vi "Close Log.vi"(0 "reference in":refnum<class "Result Logger.lvclass">, 5 "error in (no error)":errorcluster) -> (14 "reference out":refnum<class "Result Logger.lvclass">, 19 "error out":errorcluster)   [LabVIEW 2017, in "Result Logger.lvclass"]
uses:
  Result Logger.lvclass
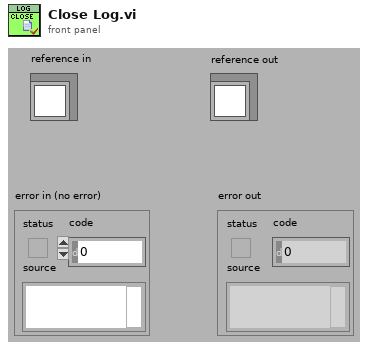
[diagram p1: front panel]
types:
  T1 = typedef "Result Logger.lvclass/ObjectAttributes.ctl" = cluster{"Logger File Path":path, "Logger File Stream":refnum<file>, "Log Messages":T2[]}
  T2 = typedef "Result Logger.lvclass/Message.ctl" = cluster{"UUT Info":cluster{"Part Number":string, "Lower Push Limit (lb)":dbl, "Upper Push Limit (lb)":dbl, "Lower Pull Limit (lb)":dbl, "Upper Pull Limit (lb)":dbl, "Push Position (mm)":dbl, "Pull Position (mm)":dbl}, "Test Results":cluster{"Test Time":timestamp, "Number of Trials":u32, "Push Values (lb)":dbl[], "Push Average (lb)":dbl, "Push Std Dev (lb)":dbl, "Push Passed":bool, "Pull Values (lb)":dbl[], "Pull Average (lb)":dbl, "Pull Std Dev (lb)":dbl, "Pull Passed":bool}}
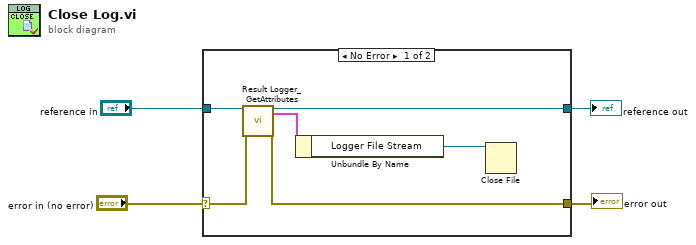
[diagram p0: block diagram]
diagram:
  n1 = case shown="No Error" "error in (no error)" {
    selector: "error in (no error)" -> [w10 w12]
    tunnel: [w8 w12] -> w3
    tunnel: [w6 w11] -> w1
    tunnel: "reference in" -> [w7 w11]
    frame No Error {
      n2 = call "Result Logger_GetAttributes.vi"("reference in"=w7, "error in (no error)"=w10) -> ("reference out"=w6:refnum<class "Result Logger.lvclass">, "Data"=w9:T1, "error out"=w8:errorcluster)  [unwired: 14 in, 1 out]
      n3 = Unbundle By Name(w9) -> ("Logger File Stream"=w5:refnum<file>)
      n4 = Close File(refnum=w5) -> ()  [unwired: 1 in, 2 out]
    }
    frame Error {
    }
  }
  "error out" <- w3
  "reference out" <- w1
